vi "Servo MSMT GSM Configure Measure Step.vi"(8 "error in (no error)":errorcluster, 10 "Standard":string="GSM", 11 "Servo MSMT in":refnum<class "Servo MSMT.lvclass">) -> (0 "error out":errorcluster, 3 "Servo MSMT out":refnum<class "Servo MSMT.lvclass">)   [LabVIEW 2018, in "Servo MSMT.lvlib" / "Servo MSMT.lvclass"]
uses:
  Servo MSMT.lvclass
  C:/Sequence Automation/Plugins/Measurement Interface.lvlibp/Measurement Interface.lvclass
  Plugins/Measurement Interface.lvlibp/Private Methods/Measurement Name/Read Measurement Name.vi
  Plugins/TestStand API Tools (TSAT).lvlibp/Step Actions/TSAT Step Actions.lvlib
  Plugins/Measurement Interface.lvlibp/Measurement Interface.lvclass
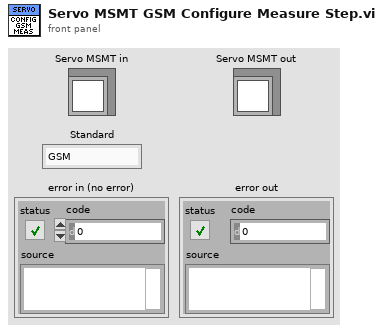
[diagram p1: front panel]
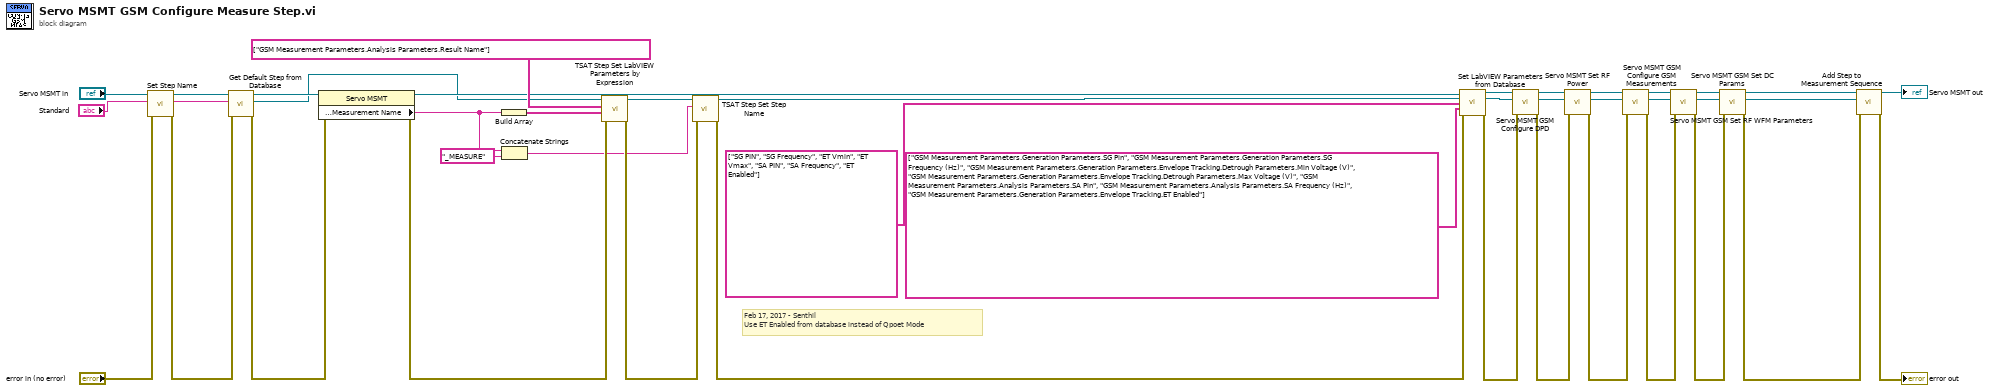
[diagram p0: block diagram]
diagram:
  # "Feb 17, 2017 - Senthil\nUse ET Enabled from database instead of Qpoet Mode"
  n1 = call-dynamic "Set Step Name.vi"("error in (no error)"="error in (no error)", "Standard"="Standard", "Servo MSMT in"="Servo MSMT in") -> ("error out"=w12:errorcluster, "Default Step"=w8:string, "Servo MSMT out"=w10:refnum<class "Servo MSMT.lvclass">)  [unwired: 6 in]
  n2 = call "Get Default Step from Database.vi"("error in (no error)"=w12, "Default Step"=w8, "Measurement Interface in"=w10) -> ("error out"=w26:errorcluster, "Cloned Step"=w24:refnum<k7>, "Measurement Interface out"=w29:refnum<class "Servo MSMT.lvclass">)  [unwired: 6 in]
  n3 = property class="Servo MSMT"(reference=w29, error in=w26) -> (reference out=w28:refnum<class "Servo MSMT.lvclass">, error out=w25:errorcluster, "Public Methods:Measurement Name"=w3:string)
  n4 = Build Array(w3) -> (w42:string[])
  n5 = Concatenate Strings(w3, "_MEASURE" ("string")) -> (w2:string)
  n6 = call "TSAT Step Set LabVIEW Parameters by Expression.vi"("Error In"=w25, "Value Expressions"=w42, "Parameters to Set"=string[] ["GSM Measurement Parameters.Analysis Parameters.Result Name"], "Step In"=w24) -> ("Error Out"=w5:errorcluster, "Step Out"=w7:refnum<k7>)  [unwired: 6 in]
  n7 = call "TSAT Step Set Step Name.vi"("Error In"=w5, "Name"=w2, "Step In"=w7) -> ("Error Out"=w4:errorcluster, "Step Out"=w6:refnum<k7>)  [unwired: 7 in]
  n8 = call "Set LabVIEW Parameters from Database.vi"("Measurement Interface in"=w28, "Step In"=w6, "Dictionary Keys"=string[] ["SG PIN", "SG Frequency", "ET Vmin", "ET Vmax", "SA PIN", "SA Frequency", "ET Enabled"] ("Database Keys"), "LabVIEW Parameter Mapping"=string[] ["GSM Measurement Parameters.Generation Parameters.SG Pin", "GSM Measurement Parameters.Generation Parameters.SG Frequency (Hz)", "GSM Measurement Parameters.Generation Parameters.Envelope Tracking.Detrough Parameters.Min Voltage (V)", "GSM Measurement Parameters.Generation Parameters.Envelope Tracking.Detrough Parameters.Max Voltage (V)", "GSM Measurement Parameters.Analysis Parameters.SA Pin", "GSM Measurement Parameters.Analysis Parameters.SA Frequency (Hz)", "GSM Measurement Parameters.Generation Parameters.Envelope Tracking.ET Enabled"] ("Database Keys"), "error in (no error)"=w4) -> ("Measurement Interface out"=w21:refnum<class "Servo MSMT.lvclass">, "Step Out"=w19:refnum<k7>, "error out"=w23:errorcluster)  [unwired: 8 in]
  n9 = call "Servo MSMT GSM Configure DPD.vi"("error in (no error)"=w23, "Step In"=w19, "Servo MSMT in"=w21) -> ("error out"=w22:errorcluster, "Step Out"=w18:refnum<k7>, "Servo MSMT out"=w20:refnum<class "Servo MSMT.lvclass">)  [unwired: 6 in]
  n10 = call-dynamic "Servo MSMT Set RF Power.vi"("error in (no error)"=w22, "Step In"=w18, "Servo MSMT in"=w20) -> ("error out"=w14:errorcluster, "Step Out"=w16:refnum<k7>, "Servo MSMT out"=w30:refnum<class "Servo MSMT.lvclass">)  [unwired: 6 in]
  n11 = call "Servo MSMT GSM Configure GSM Measurements.vi"("error in (no error)"=w14, "Step In"=w16, "Servo MSMT in"=w30) -> ("error out"=w13:errorcluster, "Step Out"=w15:refnum<k7>, "Servo MSMT out"=w17:refnum<class "Servo MSMT.lvclass">)  [unwired: 6 in]
  n12 = call "Servo MSMT GSM Set RF WFM Parameters.vi"("error in (no error)"=w13, "Step In"=w15, "Servo MSMT in"=w17) -> ("error out"=w35:errorcluster, "Step Out"=w32:refnum<k7>, "Servo MSMT out"=w37:refnum<class "Servo MSMT.lvclass">)  [unwired: 6 in]
  n13 = call "Servo MSMT GSM Set DC Params.vi"("error in (no error)"=w35, "Step In"=w32, "Servo MSMT in"=w37) -> ("error out"=w36:errorcluster, "Step Out"=w31:refnum<k7>, "Servo MSMT out"=w39:refnum<class "Servo MSMT.lvclass">)  [unwired: 6 in]
  n14 = call "Add Step to Measurement Sequence.vi"("error in (no error)"=w36, "Step to Add"=w31, "Measurement Interface in"=w39) -> ("error out"=→"error out":errorcluster, "Measurement Interface out"=→"Servo MSMT out":refnum<class "Servo MSMT.lvclass">)  [unwired: 7 in]
